vi "Initialize.vi"(8 "error in (no error)":errorcluster, 10 "Reply to":refnum<class "Result Reply Msg.lvclass">, 11 "Measure Object in":refnum<class "da Base.lvclass">) -> (0 "error out":errorcluster, 3 "Measure Object out":refnum<class "da Base.lvclass">)   [LabVIEW 2016, in "da Base.lvclass"]
uses:
  da Base.lvclass
  Da Base Messages/Result Reply Msg/Result Reply Msg.lvclass
  da Base.lvclass/da Base.ctl
  Results/Acquired Result/Acquired Result.lvclass/Acquired Result.ctl
  Write Reply to.vi
  Read Reply to.vi
  Read Name.vi
  Results/Acquired Result/Write Sender.vi
  Results/Acquired Result/Acquired Result.lvclass
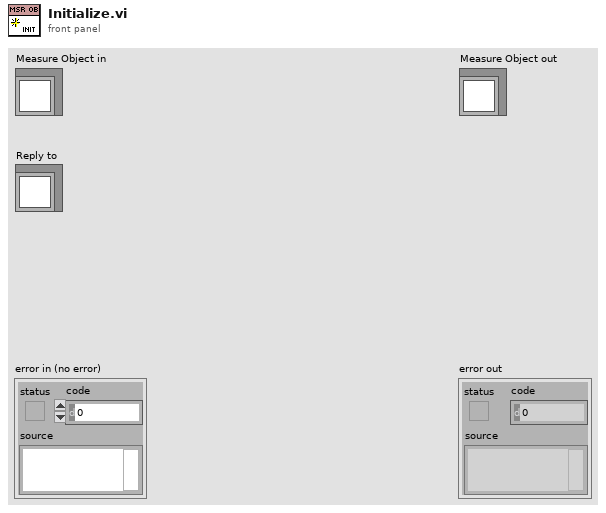
[diagram p1: front panel]
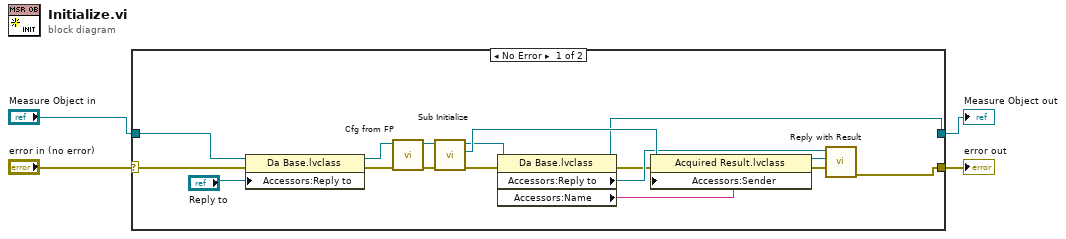
[diagram p0: block diagram]
diagram:
  n1 = case shown="No Error" "error in (no error)" {
    selector: "error in (no error)" -> [w12 w23]
    tunnel: [w21 w23] -> w3
    tunnel: [w5 w22] -> w1
    tunnel: "Measure Object in" -> [w20 w22]
    frame No Error {
      n2 = property class="Da Base.lvclass"(reference=w20, error in=w12, "Accessors:Reply to"="Reply to") -> (reference out=w14:refnum<class "da Base.lvclass">, error out=w11:errorcluster)
      n3 = call-dynamic "Cfg from FP.vi"("error in (no error)"=w11, "Measure Object in"=w14) -> ("error out"=w15:errorcluster, "Measure Object out"=w17:refnum<class "da Base.lvclass">)  [unwired: 8 in]
      n4 = call-dynamic "Sub Initialize.vi"("error in (no error)"=w15, "Measure Object in"=w17) -> ("error out"=w6:errorcluster, "Initialize Result"=w16:refnum<class "Acquired Result.lvclass">, "Measure Object out"=w10:refnum<class "da Base.lvclass">)  [unwired: 7 in]
      n5 = property class="Da Base.lvclass"(reference=w10, error in=w6) -> (reference out=w5:refnum<class "da Base.lvclass">, error out=w7:errorcluster, "Accessors:Reply to"=w8:refnum<class "Result Reply Msg.lvclass">, "Accessors:Name"=w9:string)
      n6 = property class="Acquired Result.lvclass"(reference=w16, error in=w7, "Accessors:Sender"=w9) -> (reference out=w18:refnum<class "Acquired Result.lvclass">, error out=w19:errorcluster)
      n7 = call-dynamic "Reply with Result.vi"("error in (no error)"=w19, "Result"=w18, "Result Reply Msg in"=w8) -> ("error out"=w21:errorcluster)  [unwired: 7 in, 1 out]
    }
    frame Error {
    }
  }
  "error out" <- w3
  "Measure Object out" <- w1
